vi "Demo.vi"() -> ()   [LabVIEW 2011, in "ProcessClass.lvclass"]
uses:
  ProcessClass.lvclass
panel:
  out "error out":errorcluster caption="错误输出"
  out "Process Names":string[](array[string])
  in  "停止":bool
  in  "fileName":string
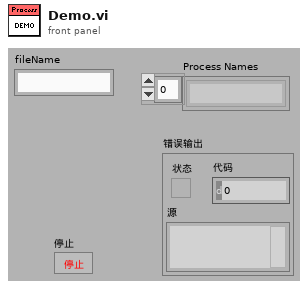
[diagram p1: front panel]
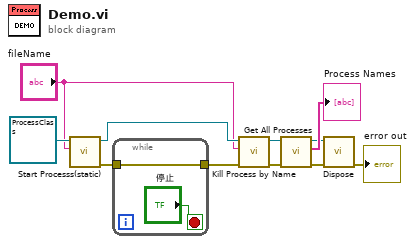
[diagram p0: block diagram]
diagram:
  n1 = call "Start Processs(static).vi"("fileName"="fileName", "ProcessClass 输入"=refnum<class "ProcessClass.lvclass"> refnum) -> ("error out"=w8:errorcluster, "ProcessClass 输出"=w10:refnum<class "ProcessClass.lvclass">)  [unwired: 7 in, 1 out]
  n2 = while {
    tunnel: w8 -> [w12]
    tunnel: [w12] -> w7
    stop <- "停止" stop-if-true
  }
  n3 = call "Kill Process by Name.vi"("error in (no error)"=w7, "processName"="fileName", "ProcessClass 输入"=w10) -> ("error out"=w5:errorcluster, "ProcessClass 输出"=w6:refnum<class "ProcessClass.lvclass">)  [unwired: 7 in]
  n4 = call "Get All Processes.vi"("error in (no error)"=w5, "ProcessClass 输入"=w6) -> ("error out"=w2:errorcluster, "Process Names"=→"Process Names":string[], "ProcessClass 输出"=w3:refnum<class "ProcessClass.lvclass">)  [unwired: 7 in]
  n5 = call "Dispose.vi"("error in (no error)"=w2, "ProcessClass 输入"=w3) -> ("error out"=→"error out":errorcluster)  [unwired: 8 in, 1 out]
